vi "Front Panel.vi"(11 "GUI In":refnum<class "GUI Composition.lvclass">) -> ()   [LabVIEW 2015, in "GUI Composition.lvclass"]
uses:
  GUI Composition.lvclass
  GUI.lvclass/GUI.ctl
  GUI Composition.lvclass/GUI Composition.ctl
  Accessors/Read RegEvent.vi
  Accessors/Read Panel Refs.vi
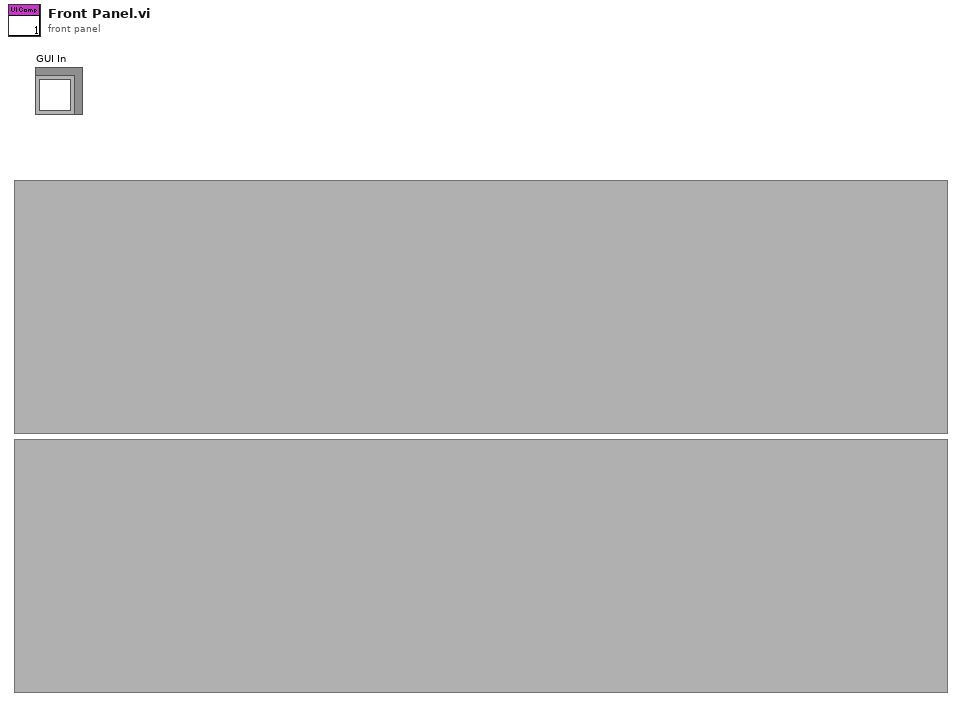
[diagram p1: front panel]
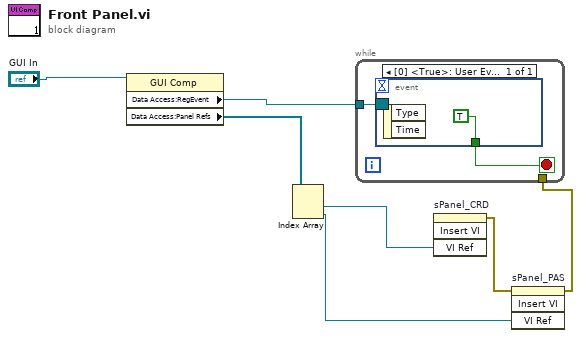
[diagram p0: block diagram]
diagram:
  n1 = property class="GUI Comp"(reference="GUI In") -> ("Data Access:RegEvent"=w6:refnum<event-registration>, "Data Access:Panel Refs"=w5:refnum<vi>[])  [unwired: 1 in, 2 out]
  n2 = Index Array(array=w5) -> (element #1=w4:refnum<vi>, element #2=w3:refnum<vi>)  [unwired: 2 in]
  n3 = invoke on="sPanel_CRD" class="SubPnl" method="Insert VI"("VI Ref"=w4) -> (error out=w2:errorcluster)  [unwired: 3 in, 3 out]
  n4 = invoke on="sPanel_PAS" class="SubPnl" method="Insert VI"(error in=w2, "VI Ref"=w3) -> (error out=w1:errorcluster)  [unwired: 2 in, 3 out]
  n5 = while {
    tunnel: w6 -> [w9]
    tunnel: w1 -> [_]
    stop <- w8 stop-if-true
    n6 = event shown="[0] <True>: User Event" {
      selector: w9 -> [_]
      dyn-events: _ -> [_]
      timeout: _ -> [_]
      tunnel: [TRUE] -> w8
      event User Event {
        n7 = event-data() -> ()  [unwired: 1 in, 2 out]
      }
    }
  }
